vi "Parse Sweep Core.vi"(0 "Scalar Path Group in":refnum<class "Scalar Path Group.lvclass">, 1 "Sweep Name":string, 5 "Config Rows":string[](array[string]), 7 "Power":dbl format="%#_13g", 9 "Frequencies":dbl[](array[numeric]), 11 "error in (no error)":errorcluster) -> (4 "Scalar Path Group out":refnum<class "Scalar Path Group.lvclass">, 15 "error out":errorcluster)   [LabVIEW 2023, in "RFFixtureCharact.Public.lvlib" / "Scalar Path Group.lvclass"]
uses:
  Scalar Path Group.lvclass
  Type Definitions/Sweep.ctl
  Common/RFCalAndFixtureCharact.Common.lvlib
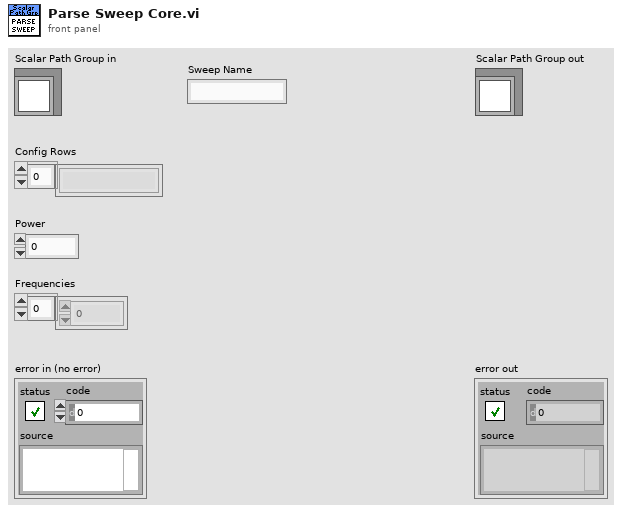
[diagram p1: front panel]
types:
  T1 = typedef "RFFixtureCharact.Public.lvlib/Scalar Path Group.lvclass/Sweep.ctl" = cluster{"Port Power":dbl, "Frequencies":dbl[], "Reference Level":dbl}
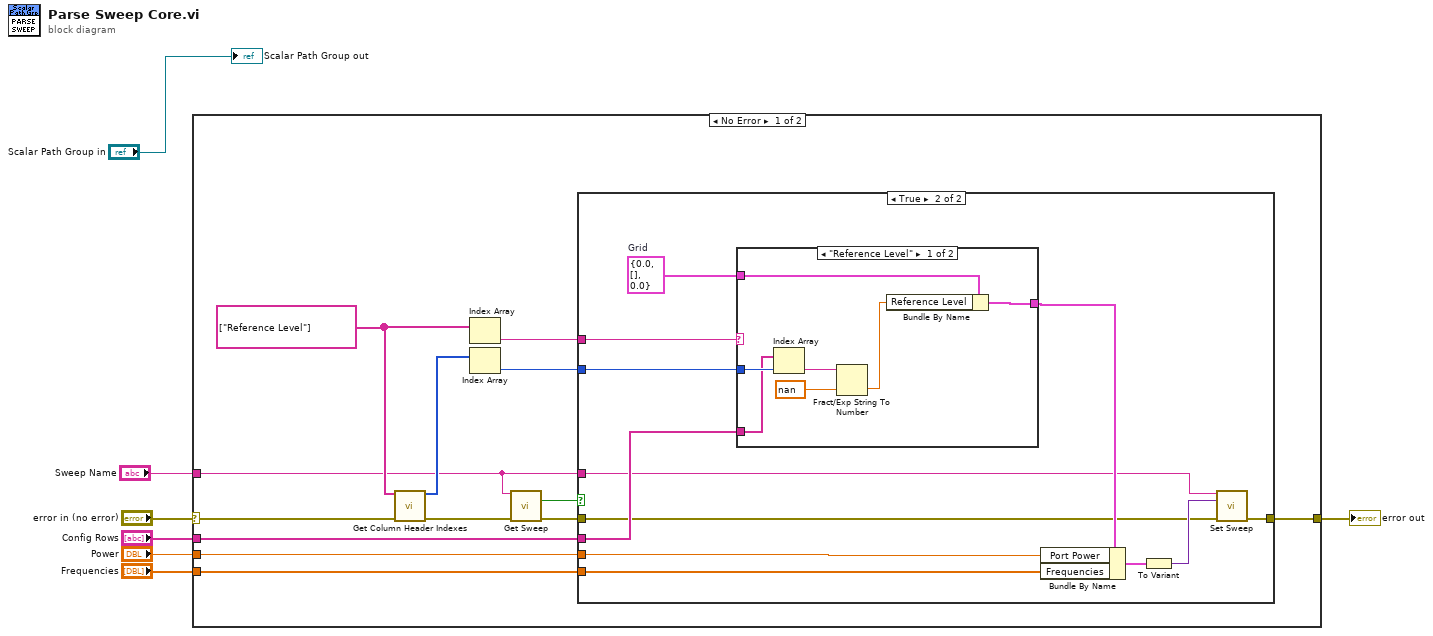
[diagram p0: block diagram]
diagram:
  n1 = case shown="No Error" "error in (no error)" {
    selector: "error in (no error)" -> [w18 w42]
    tunnel: [w20 w42] -> w4
    tunnel: "Config Rows" -> [w19 _]
    tunnel: "Power" -> [w15 _]
    tunnel: "Frequencies" -> [w14 _]
    tunnel: "Sweep Name" -> [w8 _]
    frame No Error {
      w11 = string[] ["Reference Level"] ("Column Header Names")
      n2 = call "Get Column Header Indexes.vi"("Column Header Names"=w11, "error in"=w18) -> ("Column Header Indices"=w13:i32[], "error out"=w9:errorcluster)  [unwired: 11 in, 1 out]
      n3 = Index Array(array=w11) -> (element=w10:string)  [unwired: 1 in]
      n4 = Index Array(array=w13) -> (element=w12:i32)  [unwired: 1 in]
      n5 = call "Get Sweep.vi"("Sweep Name"=w8, "error in (no error)"=w9) -> ("Sweep not found?"=w16:bool, "error out"=w17:errorcluster)  [unwired: 11 in, 1 out]
      n6 = case shown="True" w16 {
        tunnel: [w21 w33] -> w20
        tunnel: w19 -> [_ w28]
        tunnel: w17 -> [w21 w24]
        tunnel: w10 -> [_ w32]
        tunnel: w12 -> [_ w30]
        tunnel: w8 -> [_ w27]
        tunnel: w15 -> [_ w23]
        tunnel: w14 -> [_ w22]
        frame False {
        }
        frame True {
          w31 = T1 {"Port Power"=0.0, "Frequencies"=[], "Reference Level"=0.0}  # Grid
          n7 = case shown="\"Reference Level\"" w32 {
            tunnel: w31 -> [w40 w41]
            tunnel: w30 -> [w37 _]
            tunnel: [w39 w41] -> w29
            tunnel: w28 -> [w36 _]
            frame "Reference Level" {
              n8 = Index Array(array=w36, index=w37) -> (element=w35:string)
              n9 = Fract/Exp String To Number(string=w35, default (0 dbl)=nan) -> (number=w38:dbl)  [unwired: 2 in, 1 out]
              n10 = Bundle By Name(cluster=w40, "Reference Level"=w38) -> (w39:T1)
            }
            frame Default {
            }
          }
          n11 = Bundle By Name(cluster=w29, "Port Power"=w23, "Frequencies"=w22) -> (w25:T1)
          n12 = To Variant(anything=w25) -> (Variant=w26:variant)
          n13 = call "Set Sweep.vi"("Sweep Name"=w27, "Sweep in"=w26, "error in (no error)"=w24) -> ("error out"=w33:errorcluster)  [unwired: 12 in]
        }
      }
    }
    frame Error {
    }
  }
  "error out" <- w4
  "Scalar Path Group out" <- "Scalar Path Group in"
